vi "4.5.vi"() -> ()   [LabVIEW 2017]
panel:
  in  "输入":dbl
  out "次数":dbl
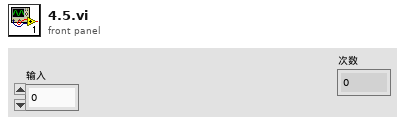
[diagram p1: front panel]
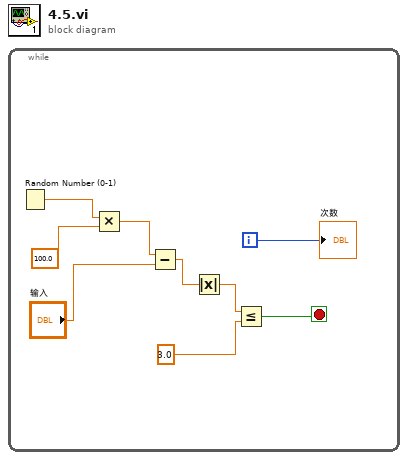
[diagram p0: block diagram]
diagram:
  n1 = while {
    i -> [w7]
    stop <- w1 stop-if-true
    n2 = Random Number (0-1)() -> (number: 0 to 1=w9:dbl)
    n3 = Multiply(x=w9, y=100.0) -> (x*y=w6:dbl)
    n4 = Subtract(x=w6, y="输入") -> (x-y=w3:dbl)
    n5 = Absolute Value(x=w3) -> (abs(x)=w2:dbl)
    n6 = Less Or Equal?(x=w2, y=3.0) -> (x <= y?=w1:bool)
    "次数" <- w7
  }
